vi "SECoP_dataGetStructCount.vi"(7 "Position":u32, 8 "error in (no error)":errorcluster, 10 "SECoP_dataPtr":T1 {"ptr64" format="%.0x"; "ptr32" format="%.0x"}, 11 "DLL path (in)":T2) -> (0 "error out":errorcluster, 2 "no. of struct elements":u32, 3 "DLL path (out)":T2)   [LabVIEW 2023, in "SECoP.lvlib"]
doc: "Call <b>\"SECoP_dataGetStructCount.vi\"</b> to access the number of possible items of a structured data type.\n\n<b>DLL path</b> input and output of cluster from \"SECoP-Initialize.vi\"\n<b>SECoP_dataPtr</b> data to access\n<b>Position</b> points to a virtual flattened entry of the data type\n<b>no. of struct elements</b> item count"
uses:
  SECoP.lvlib
  SECoP-libraries.ctl
  SECoP-data.ctl
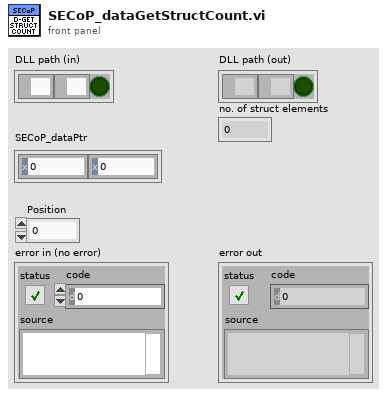
[diagram p1: front panel]
types:
  T1 = typedef "SECoP.lvlib/SECoP-data.ctl" = cluster{"ptr32":u32, "ptr64":u64}
  T2 = typedef "SECoP.lvlib/SECoP-libraries.ctl" = cluster{"serverDLL":path, "variantDLL":path, "cleanup_mode":bool}
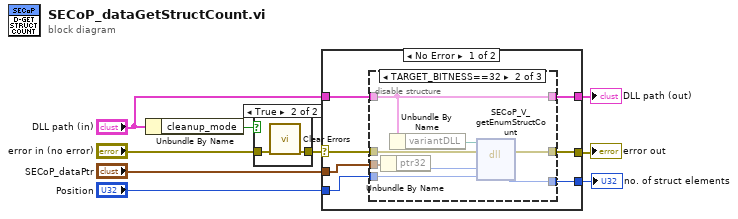
[diagram p0: block diagram]
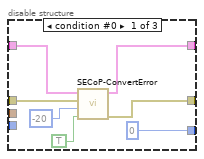
[diagram p3: hidden frame]
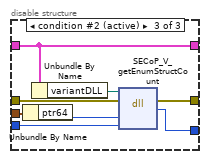
[diagram p4: hidden frame]
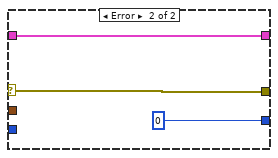
[diagram p5: hidden frame]
diagram:
  n1 = Unbundle By Name("DLL path (in)") -> ("cleanup_mode"=w6:bool)
  n2 = case shown="True" w6 {
    tunnel: "error in (no error)" -> [w10 w12]
    tunnel: [w10 w11] -> w4
    frame False {
    }
    frame True {
      n3 = call <vilib>:"Clear Errors.vi"("error in (no error)"=w12) -> ("error out"=w11:errorcluster)  [unwired: 5 in, 1 out]
    }
  }
  n4 = case shown="No Error" w4 {
    selector: w4 -> [w19 w44]
    tunnel: "DLL path (in)" -> [w18 w45]
    tunnel: [w13 w45] -> w8
    tunnel: [w16 w44] -> w7
    tunnel: "Position" -> [w17 _]
    tunnel: "SECoP_dataPtr" -> [w15 _]
    tunnel: [w14 u32 0 ("return type")] -> w1
    frame No Error {
      n5 = disable-structure shown="TARGET_BITNESS==32" {
        disable-tunnel: w19 -> [w25 w34 w42]
        disable-tunnel: w18 -> [w26 w27 w35]
        disable-tunnel: w17 -> [_ w33 w41]
        disable-tunnel: [w24 w32 w40] -> w16
        disable-tunnel: w15 -> [_ w30 w38]
        disable-tunnel: [u32 0 ("return type") w29 w37] -> w14
        disable-tunnel: [w20 w27 w35] -> w13
        frame condition #0 {
          n6 = call "SECoP-ConvertError.vi"("return is boolean"=TRUE, "return code"=-20, "error in (no error)"=w25, "DLL path (in)"=w26) -> ("error out"=w24:errorcluster, "DLL path (out)"=w20:T2)  [unwired: 6 in]
        }
        frame condition #1 {
          n7 = Unbundle By Name(w30) -> ("ptr32"=w31:u32)
          n8 = Unbundle By Name(w27) -> ("variantDLL"=w28:path)
          n9 = dll-call lib="Z:/Praktische_Aufgaben/SECoP-LabVIEW2015/32bit/SECoP32.dll" fn="SECoP_V_getEnumStructCount"(path in=w28, error in=w34, "Data"=w31, "Position"=w33) -> (error out=w32:errorcluster, "return type"=w29:u32)  [unwired: 3 in, 1 out]
        }
        frame condition #2 (active) {
          n10 = Unbundle By Name(w38) -> ("ptr64"=w39:u64)
          n11 = Unbundle By Name(w35) -> ("variantDLL"=w36:path)
          n12 = dll-call lib="Z:/Praktische_Aufgaben/SECoP-LabVIEW2015/32bit/SECoP32.dll" fn="SECoP_V_getEnumStructCount"(path in=w36, error in=w42, "Data"=w39, "Position"=w41) -> (error out=w40:errorcluster, "return type"=w37:u32)  [unwired: 3 in, 1 out]
        }
      }
    }
    frame Error {
    }
  }
  "DLL path (out)" <- w8
  "error out" <- w7
  "no. of struct elements" <- w1
